vi "Omniax_mDrive_COM9_MM_BR.vi"() -> ()   [LabVIEW 2009]
uses:
  <vilib>/Instr/_visa.llb/VISA Configure Serial Port (Instr).vi
panel:
  out "Backlash corr":bool
  in  "Y Scan set":bool
  in  "Y Scan Velocity SP mm/sec":dbl
  in  "Y Scan Length SP mm":dbl
  in  "Y Move Set":bool
  out "Backlash steps/sec":i32
  out "Backlash":i32
  out "Y in Motion":bool
  in  "Reset":bool
  out "Reset Motor Step to":dbl
  in  "Reset Y Position to":dbl
  out "Y Velocity MV mm/sec":dbl
  in  "Y Velocity SP mm/sec":dbl
  in  "Y Position SP mm":dbl
  out "Y Position MV mm":dbl
  out "Holding Current %":i32
  out "Run Current %":i32
  out "Y Scan velocity MV mm/sec":dbl format="%#_6f"
  out "Y Scan length MV mm":dbl
  in  "Y Scan Cancel":bool
  out "Y Position mm PV":dbl
  out "offset":dbl
  out "mm/rev":dbl
  out "steps/rev":u32
  out "scan steps/secm return":i32
  in  "Y Scan Length SP steps":i32 min=-460800 max=460800 step=100
  out "Y Scan":bool
  in  "Y Scan Set":bool
  in  "Scan Go":bool
  in  "Y Velocity SP step/sec":i32
  in  "Y Scan Velocity SP steps/sec":i32=1 min=1 max=102400 step=1
  in  "Stop":bool
  out "Y in Range":bool
  out "Y Step PV":i32 max=2000
  out "Status":string
  in  "Go":bool
  in  "Y Step SP":i32=-20000 min=-460800 max=460800 step=500
  out "MINPOS":i32=-94296
  out "MAXPOS":i32=-34296
  out "COM PORT":refnum<visa-resource-name>="COM5"
  # "SY"
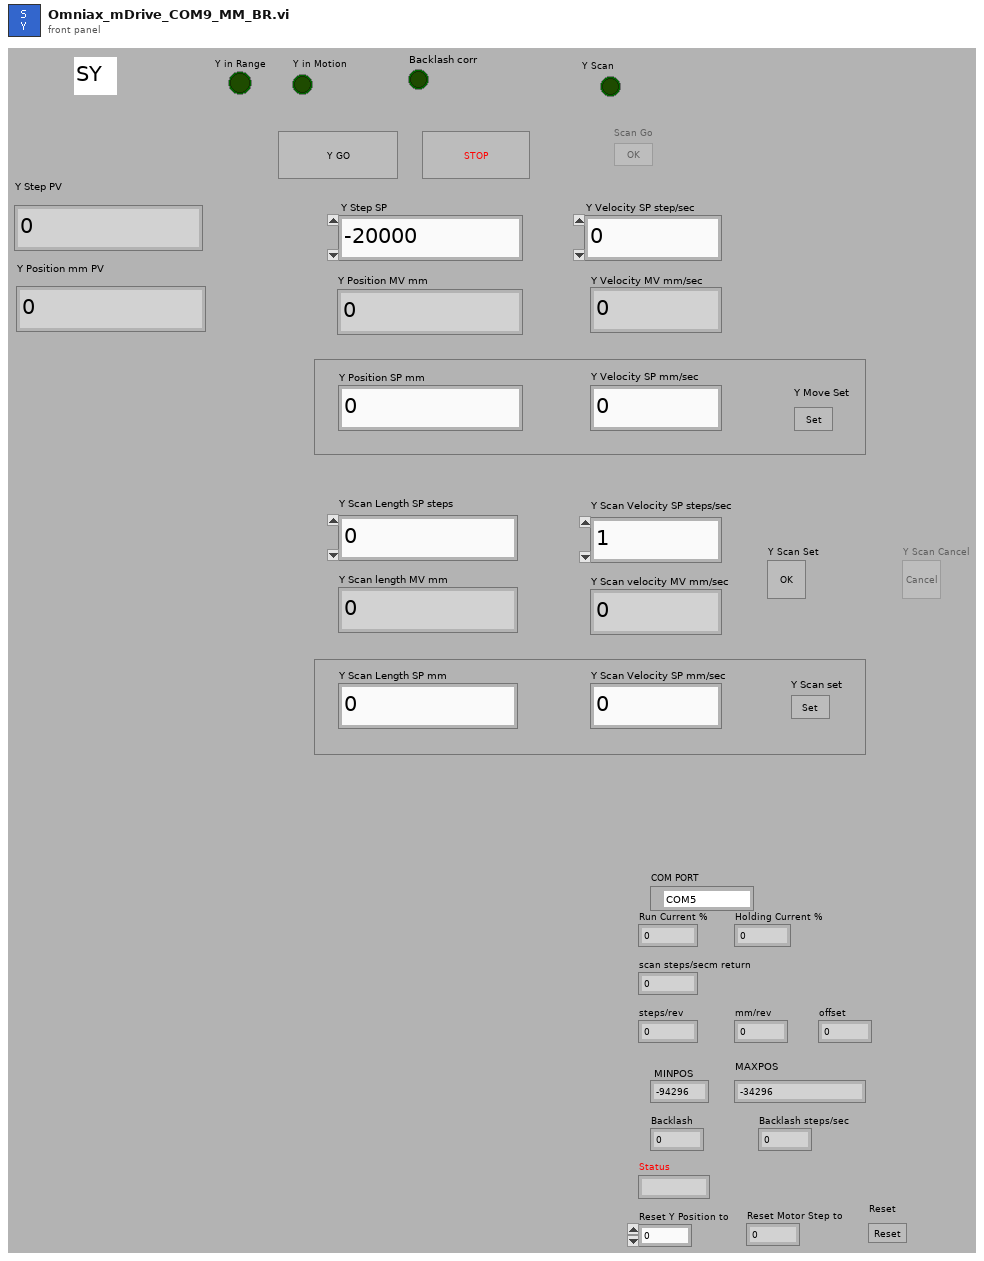
[diagram p1: front panel]
types:
  T1 = enum8{"Enabled", "Disabled", "Disabled and Grayed Out"}
  T2 = enum16{"Stop", "Reset", "Run Current", "Holding Current", "Accel Rate", "Decel Rate", "Move to Relative Position", "Move to Absolute Position", "Echo Mode", "Print Parameter", "Send String", "Microstep Resolution", "Set Current Position", "Max Velocity"}
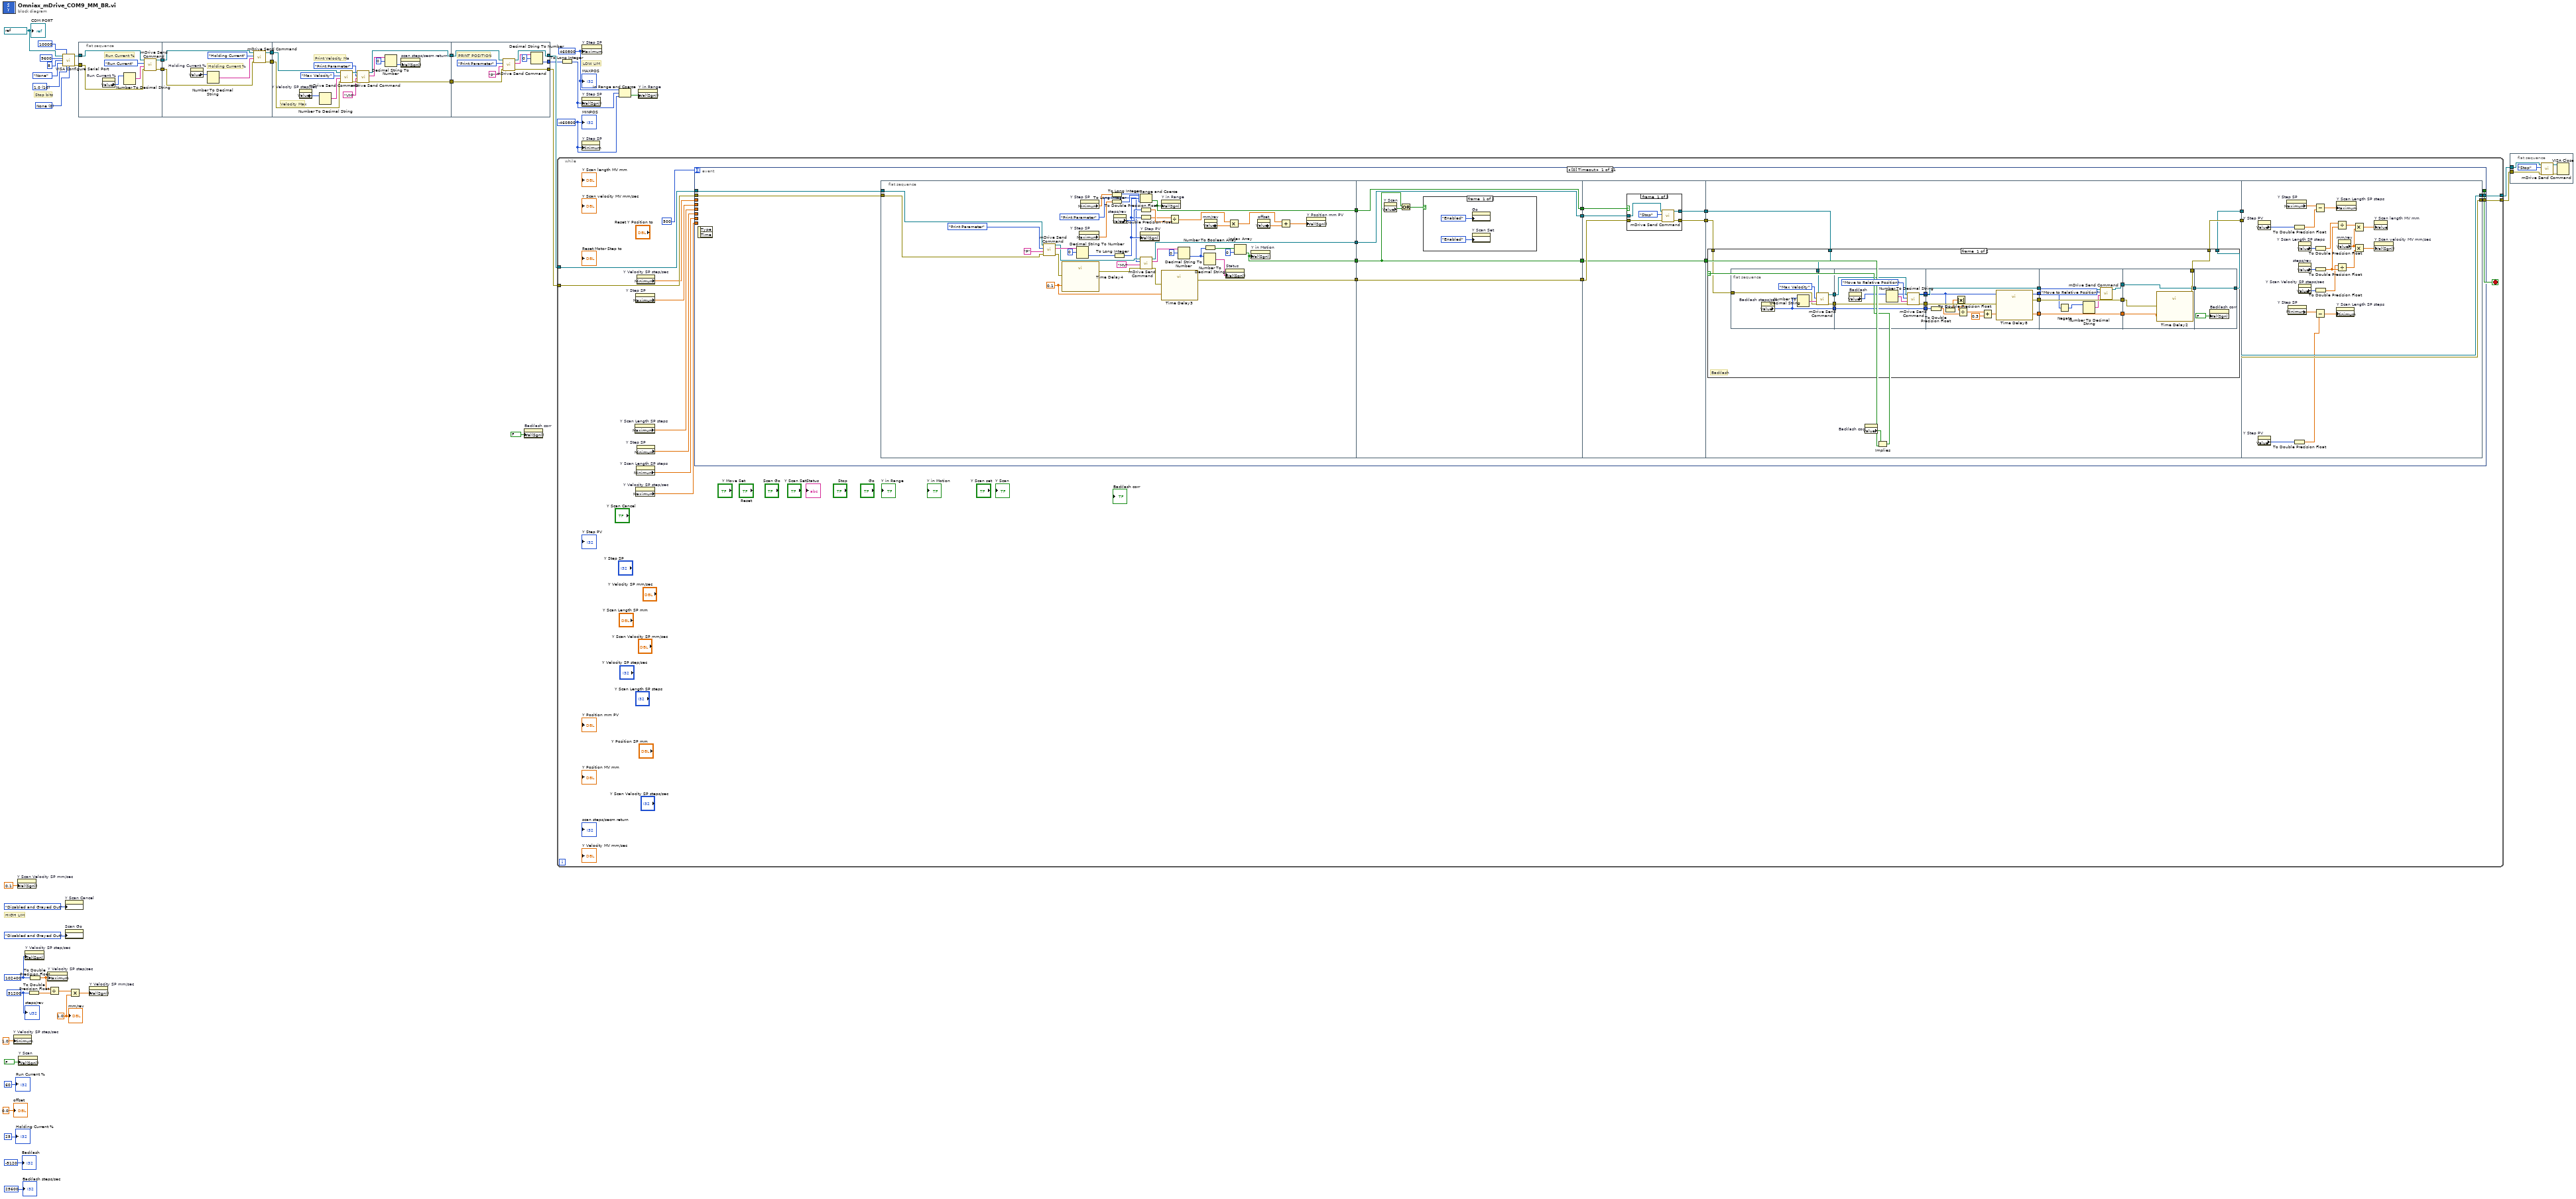
[diagram p0: block diagram]
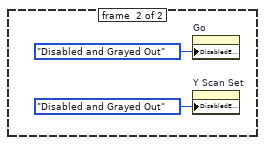
[diagram p2: hidden frame]
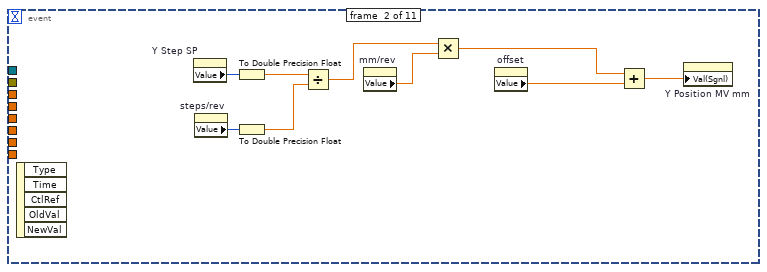
[diagram p5: hidden frame]
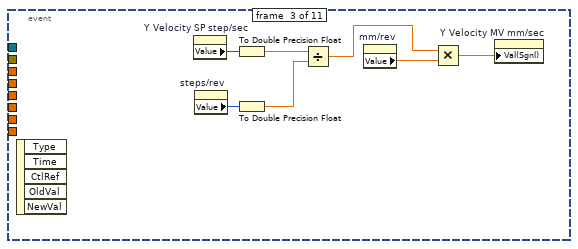
[diagram p6: hidden frame]
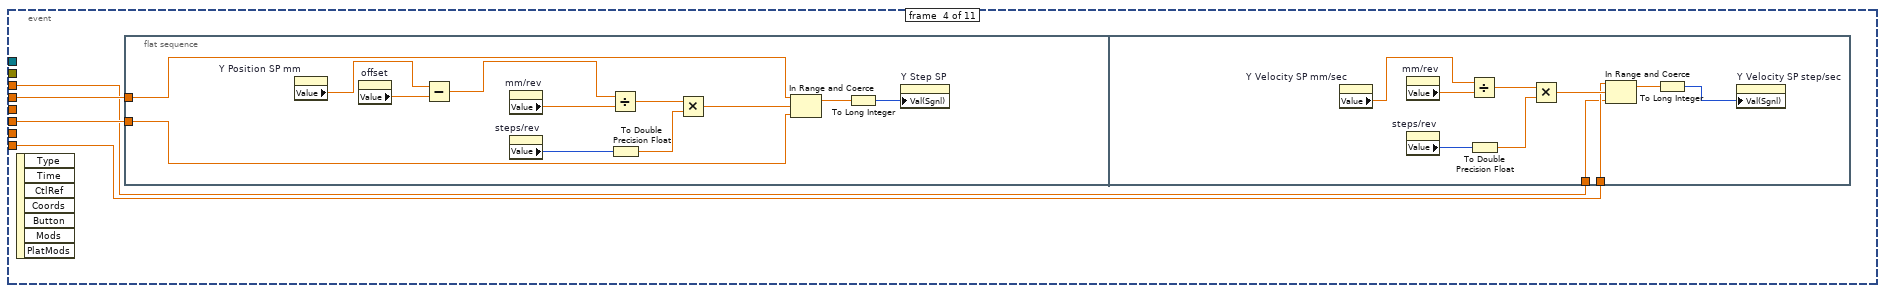
[diagram p7: hidden frame]
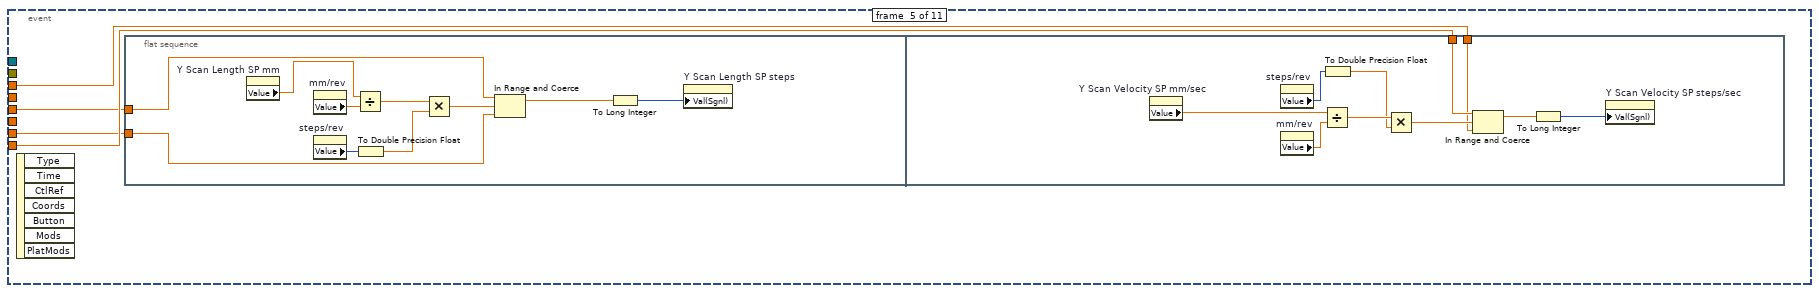
[diagram p8: hidden frame]
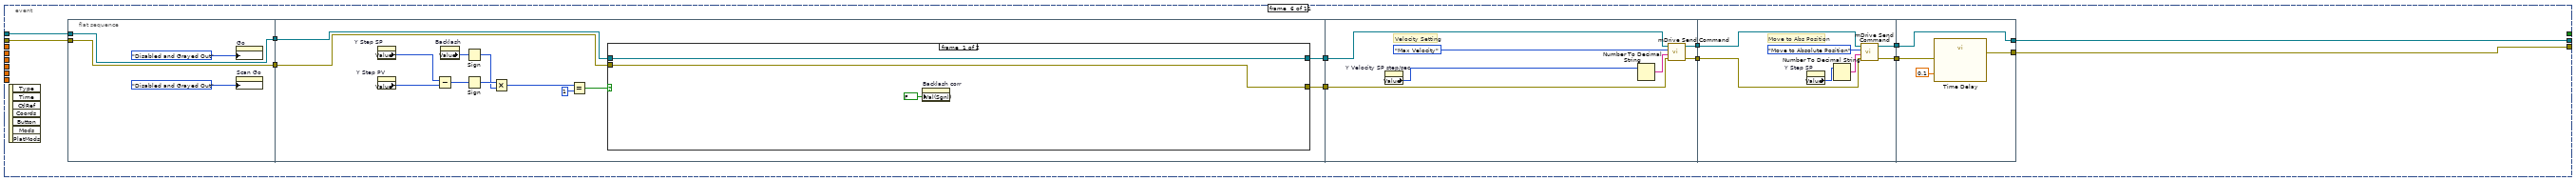
[diagram p9: hidden frame]
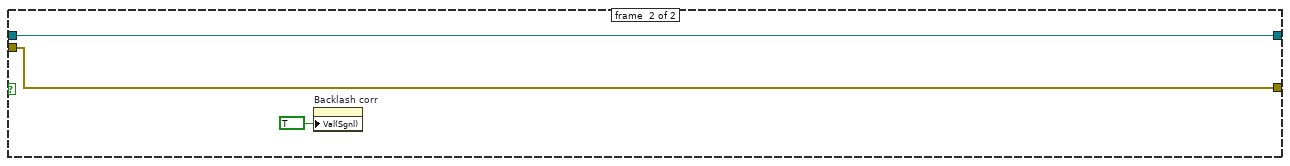
[diagram p10: hidden frame]
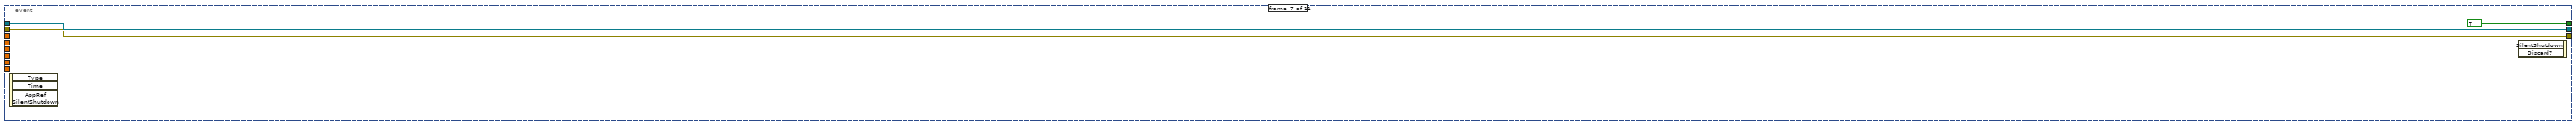
[diagram p11: hidden frame]
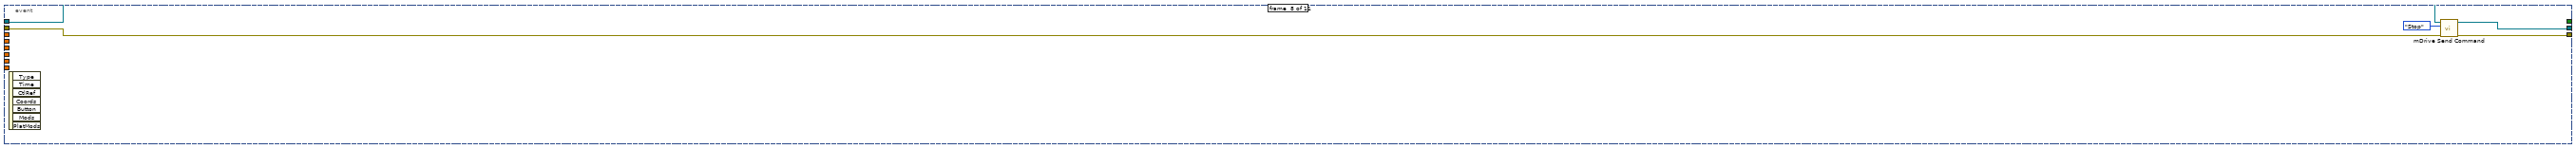
[diagram p12: hidden frame]
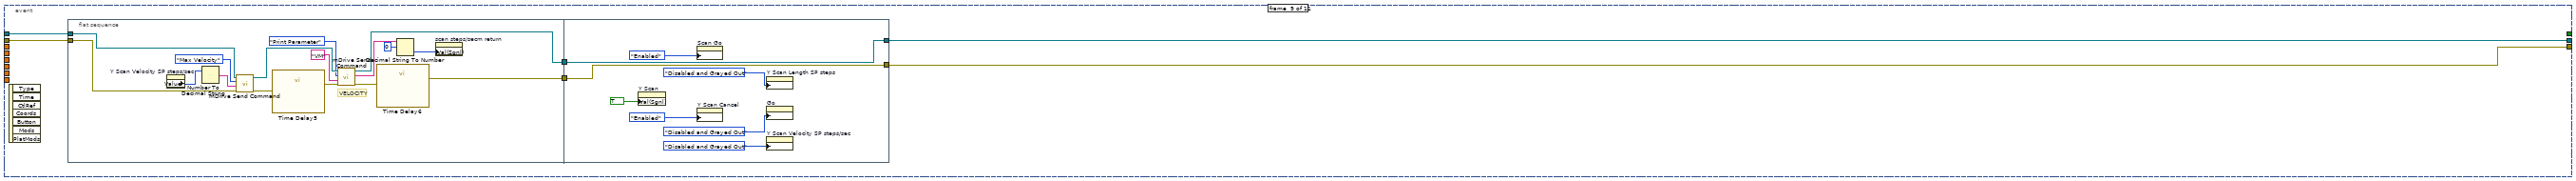
[diagram p13: hidden frame]
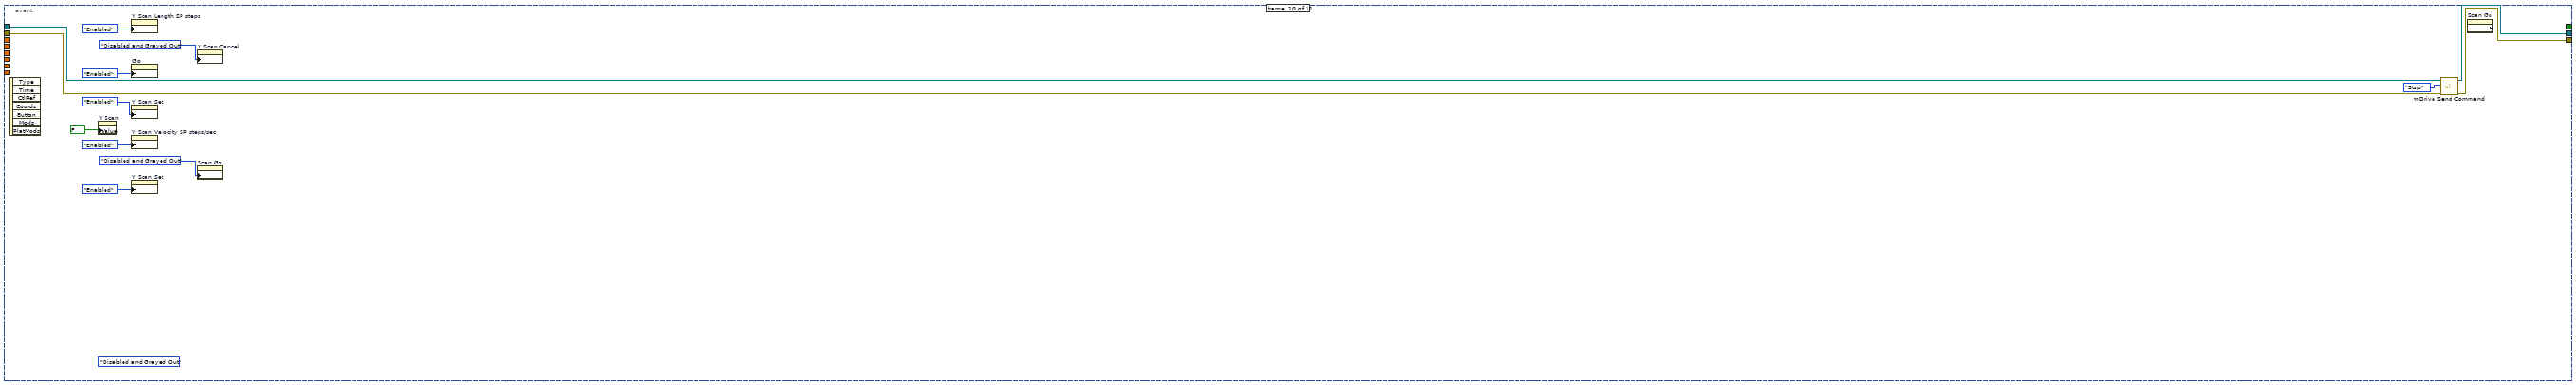
[diagram p14: hidden frame]
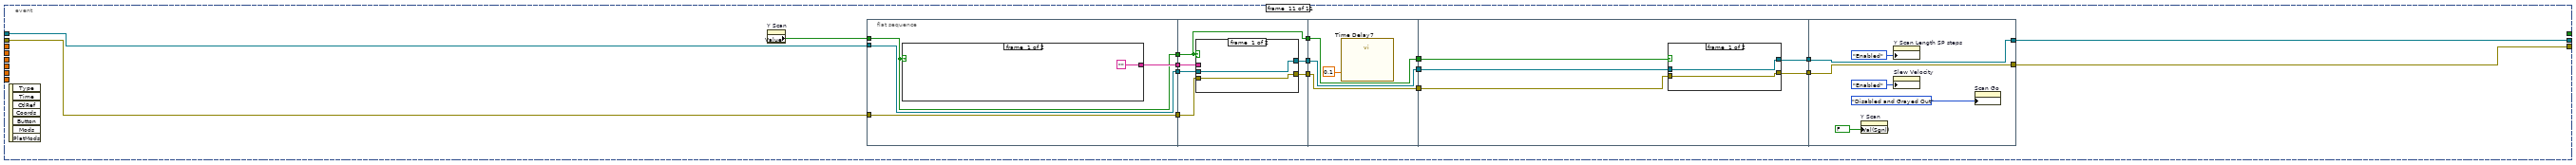
[diagram p15: hidden frame]
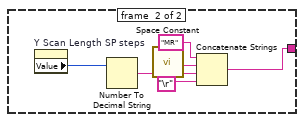
[diagram p16: hidden frame]
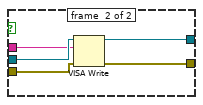
[diagram p17: hidden frame]
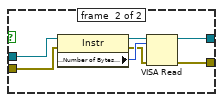
[diagram p18: hidden frame]
diagram:
  w7 = 1.0 ("MM/rev")
  w4 = u32 51200 ("step/rev")
  w9 = 102400 ("Value (Signaling)")
  w29 = -460800 ("lower limit")
  w28 = 460800 ("upper limit")
  w36 = refnum<visa-resource-name> "COM9" ("COM PORT")
  w38 = u16 0 items=["None", "XON/XOFF", "RTS/CTS", "XON/XOFF & RTS/CTS", "DTR/DSR", "XON/XOFF & DTR/DSR"] ("flow control (0:none)")
  w39 = u16 10 items=["1.0"=10, "1.5"=15, "2.0"=20] ("stop bits (10: 1 bit)")
  # "HIGH LIM"
  # "LOW LIM"
  # "Stop bits"
  n1 = property on="Y Velocity SP step/sec" class="DigNum (strict)"("Minimum"=1.0 ("Data Entry Limits:Minimum")) -> ()  [unwired: 2 in, 2 out]
  n2 = property on="Y Scan Velocity SP mm/sec" class="DigNum (strict)"("Val(Sgnl)"=0.1 ("Value (Signaling)")) -> ()  [unwired: 2 in, 2 out]
  n3 = property on="Y Scan" class="Bool (strict)"("Val(Sgnl)"=FALSE ("Value (Signaling)")) -> ()  [unwired: 2 in, 2 out]
  n4 = property on="Y Velocity SP step/sec" class="DigNum (strict)"("Val(Sgnl)"=w9) -> ()  [unwired: 2 in, 2 out]
  n5 = To Double Precision Float(number=w4) -> (double precision float=w5:dbl)
  n6 = To Double Precision Float(number=w9) -> (double precision float=w3:dbl)
  n7 = property on="Y Velocity SP step/sec" class="DigNum (strict)"("Maximum"=w3) -> ()  [unwired: 2 in, 2 out]
  n8 = Divide(x=w3, y=w5) -> (x/y=w8:dbl)
  n9 = call-poly "VISA Configure Serial Port"("VISA resource name"=w36, "timeout (10sec)"=u32 10000, "baud rate (9600)"=u32 9600, "data bits (8)"=u16 8, "parity (0:none)"=enum16{"None", "Odd", "Even", "Mark", "Space"}."None", "stop bits (10: 1 bit)"=w39, "flow control (0:none)"=w38) -> ("VISA resource name out"=w24:refnum<visa-resource-name>, "error out"=w23:errorcluster)  [unwired: 7 in]
  n10 = property on="Y Scan Cancel" class="Bool"("DisabledEnum"=T1."Disabled and Grayed Out" ("Disabled")) -> ()  [unwired: 2 in, 2 out]
  n11 = property on="Scan Go" class="Bool"("DisabledEnum"=T1."Disabled and Grayed Out" ("Disabled")) -> ()  [unwired: 2 in, 2 out]
  n12 = Multiply(x=w8, y=w7) -> (x*y=w6:dbl)
  n13 = flat-sequence {
    tunnel: w23 -> [w49]
    tunnel: w24 -> [w47]
    tunnel: [w46] -> w18
    tunnel: [w48] -> w16
    tunnel: w18 -> [w56]
    tunnel: [w55] -> w17
    tunnel: w16 -> [w53]
    tunnel: [w54] -> w15
    tunnel: [w66] -> w26
    tunnel: [w67] -> w25
    tunnel: w17 -> [w65]
    tunnel: w15 -> [w64]
    tunnel: [w79] -> w35
    tunnel: [w78] -> w34
    tunnel: [w73] -> w27
    tunnel: w26 -> [w77]
    tunnel: w25 -> [w76]
    frame #0 {
      # "Run Current %"
      n14 = property on="Run Current %" class="DigNum (strict)"() -> ("Value"=w44:i32)  [unwired: 2 in, 2 out]
      n15 = Number To Decimal String(number=w44) -> (decimal integer string=w45:string)  [unwired: 1 in]
      n16 = call "mDrive Send Command.vi"("error in (no error)"=w49, "Extra"=w45, "Command"=T2."Run Current", "VISA resource name"=w47) -> ("error out"=w48:errorcluster, "VISA resource name out"=w46:refnum<visa-resource-name>)  [unwired: 3 in, 1 out]
    }
    frame #1 {
      # "Holding Current %"
      n17 = property on="Holding Current %" class="DigNum (strict)"() -> ("Value"=w51:i32)  [unwired: 2 in, 2 out]
      n18 = Number To Decimal String(number=w51) -> (decimal integer string=w52:string)  [unwired: 1 in]
      n19 = call "mDrive Send Command.vi"("error in (no error)"=w53, "Extra"=w52, "Command"=T2."Holding Current", "VISA resource name"=w56) -> ("error out"=w54:errorcluster, "VISA resource name out"=w55:refnum<visa-resource-name>)  [unwired: 3 in, 1 out]
    }
    frame #2 {
      # "Print Velocity Ma"
      # "Velocity Max"
      n20 = property on="Y Velocity SP step/sec" class="DigNum (strict)"() -> ("Value"=w63:i32)  [unwired: 2 in, 2 out]
      n21 = Number To Decimal String(number=w63) -> (decimal integer string=w62:string)  [unwired: 1 in]
      n22 = call "mDrive Send Command.vi"("error in (no error)"=w64, "Extra"=w62, "Command"=T2."Max Velocity", "VISA resource name"=w65) -> ("error out"=w60:errorcluster, "VISA resource name out"=w70:refnum<visa-resource-name>)  [unwired: 3 in, 1 out]
      n23 = call "mDrive Send Command.vi"("error in (no error)"=w60, "Extra"="VM", "Command"=T2."Print Parameter", "VISA resource name"=w70) -> ("error out"=w67:errorcluster, "read buffer"=w68:string, "VISA resource name out"=w66:refnum<visa-resource-name>)  [unwired: 3 in]
      n24 = Decimal String To Number(string=w68, offset=0) -> (number=w61:i32)  [unwired: 1 in, 1 out]
      n25 = property on="scan steps/secm return" class="DigNum (strict)"("Val(Sgnl)"=w61) -> ()  [unwired: 2 in, 2 out]
    }
    frame #3 {
      # "PRINT POSITION"
      n26 = call "mDrive Send Command.vi"("error in (no error)"=w76, "Extra"="P", "Command"=T2."Print Parameter", "VISA resource name"=w77) -> ("error out"=w78:errorcluster, "read buffer"=w75:string, "VISA resource name out"=w79:refnum<visa-resource-name>)  [unwired: 3 in]
      n27 = Decimal String To Number(string=w75, offset=0) -> (number=w73:i32)  [unwired: 1 in, 1 out]
    }
  }
  n28 = property on="Y Velocity SP mm/sec" class="DigNum (strict)"("Val(Sgnl)"=w6) -> ()  [unwired: 2 in, 2 out]
  n29 = property on="Backlash corr" class="Bool (strict)"("Val(Sgnl)"=FALSE ("Value (Signaling)")) -> ()  [unwired: 2 in, 2 out]
  n30 = while {
    tunnel: w35 -> [w87]
    tunnel: w34 -> [w90]
    tunnel: [w91] -> w31
    tunnel: [w89] -> w32
    stop <- w86 stop-if-true
    n31 = property on="Y Scan Length SP steps" class="DigNum (strict)"() -> ("Maximum"=w80:dbl)  [unwired: 2 in, 2 out]
    n32 = property on="Y Step SP" class="DigNum (strict)"() -> ("Maximum"=w84:dbl)  [unwired: 2 in, 2 out]
    n33 = property on="Y Velocity SP step/sec" class="DigNum (strict)"() -> ("Maximum"=w83:dbl)  [unwired: 2 in, 2 out]
    n34 = property on="Y Scan Length SP steps" class="DigNum (strict)"() -> ("Minimum"=w81:dbl)  [unwired: 2 in, 2 out]
    n35 = property on="Y Velocity SP step/sec" class="DigNum (strict)"() -> ("Minimum"=w82:dbl)  [unwired: 2 in, 2 out]
    n36 = property on="Y Step SP" class="DigNum (strict)"() -> ("Minimum"=w85:dbl)  [unwired: 2 in, 2 out]
    n37 = event shown="[0] Timeout" {
      selector: _ -> [_ _ _ _ _ _ _ _ _ _ _]
      dyn-events: _ -> [_ _ _ _ _ _ _ _ _ _ _]
      timeout: 500 -> [_ _ _ _ _ _ _ _ _ _ _]
      tunnel: w90 -> [w108 _ _ _ _ w328 w378 w383 w390 w420 w444]
      tunnel: [w107 _ _ _ _ w334 w378 w381 w388 w422 w441] -> w91
      tunnel: w87 -> [w105 _ _ _ _ w329 w379 w384 w389 w421 w443]
      tunnel: [w106 _ _ _ _ w335 w379 w382 w385 w423 w442] -> w89
      tunnel: [_ _ _ _ _ _ TRUE _ _ _ _] -> w86
      tunnel: w85 -> [_ _ _ w277 _ _ _ _ _ _ _]
      tunnel: w84 -> [_ _ _ w276 _ _ _ _ _ _ _]
      tunnel: w83 -> [_ _ _ w275 w303 _ _ _ _ _ _]
      tunnel: w82 -> [_ _ _ w274 w302 _ _ _ _ _ _]
      tunnel: w81 -> [_ _ _ _ w301 _ _ _ _ _ _]
      tunnel: w80 -> [_ _ _ _ w300 _ _ _ _ _ _]
      event #0 {
        n38 = event-data() -> ()  [unwired: 1 in, 2 out]
        n39 = flat-sequence {
          tunnel: w108 -> [w140]
          tunnel: w105 -> [w139]
          tunnel: [w145] -> w104
          tunnel: [w119] -> w102
          tunnel: [w132] -> w100
          tunnel: [w109] -> w98
          tunnel: w104 -> [w151]
          tunnel: [w151] -> w103
          tunnel: w102 -> [w150]
          tunnel: [w150] -> w101
          tunnel: w100 -> [w149]
          tunnel: [w149] -> w99
          tunnel: w98 -> [w146]
          tunnel: [w146] -> w93
          tunnel: w103 -> [w158]
          tunnel: [w159] -> w97
          tunnel: w101 -> [w161]
          tunnel: [w160] -> w96
          tunnel: w99 -> [w157]
          tunnel: [w156] -> w94
          tunnel: w93 -> [w156]
          tunnel: w97 -> [w171]
          tunnel: w96 -> [w172]
          tunnel: [w170] -> w95
          tunnel: w94 -> [w174]
          tunnel: [w169] -> w92
          tunnel: [w256] -> w107
          tunnel: [w257] -> w106
          tunnel: w95 -> [w256]
          tunnel: w92 -> [w257]
          frame #0 {
            w113 = 0.1 ("Delay Time (s)")
            n40 = call "mDrive Send Command.vi"("error in (no error)"=w140, "Extra"="P", "Command"=T2."Print Parameter", "VISA resource name"=w139) -> ("error out"=w138:errorcluster, "read buffer"=w144:string, "VISA resource name out"=w142:refnum<visa-resource-name>)  [unwired: 3 in]
            n41 = call "Time Delay4"("error in (no error)"=w138, "Delay Time (s)"=w113) -> ("error out"=w137:errorcluster)  [unwired: 9 in]
            n42 = Decimal String To Number(string=w144, offset=0) -> (number=w122:i32)  [unwired: 1 in, 1 out]
            n43 = property on="Y Step SP" class="DigNum (strict)"() -> ("Maximum"=w134:dbl)  [unwired: 2 in, 2 out]
            n44 = property on="Y Step SP" class="DigNum (strict)"() -> ("Minimum"=w136:dbl)  [unwired: 2 in, 2 out]
            n45 = To Long Integer(number=w136) -> (32bit integer=w135:i32)
            n46 = To Long Integer(number=w134) -> (32bit integer=w133:i32)
            n47 = To Long Integer(number=w122) -> (32bit integer=w124:i32)
            n48 = property on="steps/rev" class="DigNum (strict)"() -> ("Value"=w130:u32)  [unwired: 2 in, 2 out]
            n49 = In Range and Coerce(upper limit=w133, x=w124, lower limit=w135) -> (In Range?=w132:bool)  [unwired: 1 out]
            n50 = To Double Precision Float(number=w130) -> (double precision float=w131:dbl)
            n51 = To Double Precision Float(number=w124) -> (double precision float=w125:dbl)
            n52 = property on="Y Step PV" class="DigNum (strict)"("Val(Sgnl)"=w124) -> ()  [unwired: 2 in, 2 out]
            n53 = call "mDrive Send Command.vi"("error in (no error)"=w137, "Extra"="MV", "Command"=T2."Print Parameter", "VISA resource name"=w142) -> ("error out"=w141:errorcluster, "read buffer"=w120:string, "VISA resource name out"=w145:refnum<visa-resource-name>)  [unwired: 3 in]
            n54 = property on="Y in Range" class="Bool (strict)"("Val(Sgnl)"=w132) -> ()  [unwired: 2 in, 2 out]
            n55 = call "Time Delay3"("error in (no error)"=w141, "Delay Time (s)"=w113) -> ("error out"=w119:errorcluster)  [unwired: 9 in]
            n56 = Divide(x=w125, y=w131) -> (x/y=w129:dbl)
            n57 = Decimal String To Number(string=w120, offset=0 ("offset (0)")) -> (number=w112:i32)  [unwired: 1 in, 1 out]
            n58 = Number To Decimal String(number=w112) -> (decimal integer string=w118:string)  [unwired: 1 in]
            n59 = property on="mm/rev" class="DigNum (strict)"() -> ("Value"=w128:dbl)  [unwired: 2 in, 2 out]
            n60 = Number To Boolean Array(number=w112) -> (Boolean array=w111:bool[])
            n61 = property on="Status" class="Str"("Val(Sgnl)"=w118) -> ()  [unwired: 2 in, 2 out]
            n62 = Multiply(x=w129, y=w128) -> (x*y=w127:dbl)
            n63 = Index Array(array=w111, index=0) -> (element=w109:bool)
            n64 = property on="Y in Motion" class="Bool (strict)"("Val(Sgnl)"=w109) -> ()  [unwired: 2 in, 2 out]
            n65 = property on="offset" class="DigNum (strict)"() -> ("Value"=w126:dbl)  [unwired: 2 in, 2 out]
            n66 = Add(x=w127, y=w126) -> (x+y=w123:dbl)
            n67 = property on="Y Position mm PV" class="DigNum (strict)"("Val(Sgnl)"=w123) -> ()  [unwired: 2 in, 2 out]
          }
          frame #1 {
            n68 = property on="Y Scan" class="Bool (strict)"() -> ("Value"=w147:bool)  [unwired: 2 in, 2 out]
            n69 = Or(x=w146, y=w147) -> (x .or. y?=w148:bool)
            n70 = case shown="False" w148 {
              frame #0 {
                n71 = property on="Go" class="Bool"("DisabledEnum"=T1."Enabled" ("Disabled")) -> ()  [unwired: 2 in, 2 out]
                n72 = property on="Y Scan Set" class="Bool"("DisabledEnum"=T1."Enabled" ("Disabled")) -> ()  [unwired: 2 in, 2 out]
              }
              frame #1 {
                n73 = property on="Go" class="Bool"("DisabledEnum"=T1."Disabled and Grayed Out" ("Disabled")) -> ()  [unwired: 2 in, 2 out]
                n74 = property on="Y Scan Set" class="Bool"("DisabledEnum"=T1."Disabled and Grayed Out" ("Disabled")) -> ()  [unwired: 2 in, 2 out]
              }
            }
          }
          frame #2 {
            n75 = case shown="False" w157 {
              tunnel: w158 -> [w164 w168]
              tunnel: [w165 w168] -> w159
              tunnel: [w166 w167] -> w160
              tunnel: w161 -> [w163 w167]
              frame #0 {
                n76 = call "mDrive Send Command.vi"("error in (no error)"=w163, "Command"=T2."Stop", "VISA resource name"=w164) -> ("error out"=w166:errorcluster, "VISA resource name out"=w165:refnum<visa-resource-name>)  [unwired: 4 in, 1 out]
              }
              frame #1 {
              }
            }
          }
          frame #3 {
            n77 = property on="Backlash corr" class="Bool (strict)"() -> ("Value"=w175:bool)  [unwired: 2 in, 2 out]
            n78 = Implies(1:w174, 2:w175) -> (0:w173:bool)
            n79 = case shown="False" w173 {
              tunnel: w172 -> [w182 w235]
              tunnel: w171 -> [w181 w236]
              tunnel: [w180 w235] -> w170
              tunnel: [w179 w236] -> w169
              frame #0 {
                # "Backlash"
                n80 = flat-sequence {
                  tunnel: [w197] -> w194
                  tunnel: [w199] -> w193
                  tunnel: [w198] -> w192
                  tunnel: w182 -> [w196]
                  tunnel: w181 -> [w195]
                  tunnel: w194 -> [w207]
                  tunnel: [w207] -> w191
                  tunnel: w193 -> [w206]
                  tunnel: w192 -> [w205]
                  tunnel: [w204] -> w190
                  tunnel: [w203] -> w189
                  tunnel: [w202] -> w178
                  tunnel: w191 -> [w217]
                  tunnel: w190 -> [w216]
                  tunnel: w189 -> [w214]
                  tunnel: [w215] -> w188
                  tunnel: [w214] -> w187
                  tunnel: [w213] -> w184
                  tunnel: [w212] -> w183
                  tunnel: w178 -> [w212]
                  tunnel: w188 -> [w228]
                  tunnel: w187 -> [w221]
                  tunnel: [w228] -> w186
                  tunnel: [w227] -> w185
                  tunnel: w184 -> [w227]
                  tunnel: w183 -> [w223]
                  tunnel: [w222] -> w176
                  tunnel: w186 -> [w232]
                  tunnel: w185 -> [w231]
                  tunnel: [w230] -> w180
                  tunnel: [w229] -> w177
                  tunnel: w176 -> [w229]
                  tunnel: [w234] -> w179
                  tunnel: w177 -> [w234]
                  frame #0 {
                    n81 = property on="Backlash steps/sec" class="DigNum (strict)"() -> ("Value"=w197:i32)  [unwired: 2 in, 2 out]
                    n82 = Number To Decimal String(number=w197) -> (decimal integer string=w200:string)  [unwired: 1 in]
                    n83 = call "mDrive Send Command.vi"("error in (no error)"=w196, "Extra"=w200, "Command"=T2."Max Velocity", "VISA resource name"=w195) -> ("error out"=w198:errorcluster, "VISA resource name out"=w199:refnum<visa-resource-name>)  [unwired: 3 in, 1 out]
                  }
                  frame #1 {
                    n84 = property on="Backlash" class="DigNum (strict)"() -> ("Value"=w202:i32)  [unwired: 2 in, 2 out]
                    n85 = Number To Decimal String(number=w202) -> (decimal integer string=w208:string)  [unwired: 1 in]
                    n86 = call "mDrive Send Command.vi"("error in (no error)"=w205, "Extra"=w208, "Command"=T2."Move to Relative Position", "VISA resource name"=w206) -> ("error out"=w204:errorcluster, "VISA resource name out"=w203:refnum<visa-resource-name>)  [unwired: 3 in, 1 out]
                  }
                  frame #2 {
                    n87 = To Double Precision Float(number=w217) -> (double precision float=w219:dbl)
                    n88 = To Double Precision Float(number=w212) -> (double precision float=w210:dbl)
                    n89 = Absolute Value(x=w210) -> (abs(x)=w211:dbl)
                    n90 = Divide(x=w211, y=w219) -> (x/y=w220:dbl)
                    n91 = Add(x=w220, y=0.3) -> (x+y=w213:dbl)
                    n92 = call "Time Delay8"("error in (no error)"=w216, "Delay Time (s)"=w213) -> ("error out"=w215:errorcluster)  [unwired: 9 in]
                  }
                  frame #3 {
                    n93 = Negate(x=w223) -> (-x=w224:i32)
                    n94 = Number To Decimal String(number=w224) -> (decimal integer string=w225:string)  [unwired: 1 in]
                    n95 = call "mDrive Send Command.vi"("Extra"=w225, "Command"=T2."Move to Relative Position", "VISA resource name"=w221) -> ("VISA resource name out"=w222:refnum<visa-resource-name>)  [unwired: 4 in, 2 out]
                  }
                  frame #4 {
                    n96 = call "Time Delay2"("error in (no error)"=w232, "Delay Time (s)"=w231) -> ("error out"=w230:errorcluster)  [unwired: 9 in]
                  }
                  frame #5 {
                    n97 = property on="Backlash corr" class="Bool (strict)"("Val(Sgnl)"=FALSE ("Value (Signaling)")) -> ()  [unwired: 2 in, 2 out]
                  }
                }
              }
              frame #1 {
              }
            }
          }
          frame #4 {
            n98 = property on="Y Step PV" class="DigNum (strict)"() -> ("Value"=w246:i32)  [unwired: 2 in, 2 out]
            n99 = property on="Y Step PV" class="DigNum (strict)"() -> ("Value"=w244:i32)  [unwired: 2 in, 2 out]
            n100 = property on="Y Step SP" class="DigNum (strict)"() -> ("Maximum"=w253:dbl)  [unwired: 2 in, 2 out]
            n101 = property on="Y Step SP" class="DigNum (strict)"() -> ("Minimum"=w254:dbl)  [unwired: 2 in, 2 out]
            n102 = To Double Precision Float(number=w246) -> (double precision float=w245:dbl)
            n103 = To Double Precision Float(number=w244) -> (double precision float=w243:dbl)
            n104 = property on="Y Scan Velocity SP steps/sec" class="DigNum (strict)"() -> ("Value"=w241:i32)  [unwired: 2 in, 2 out]
            n105 = property on="Y Scan Length SP steps" class="DigNum (strict)"() -> ("Value"=w250:i32)  [unwired: 2 in, 2 out]
            n106 = property on="steps/rev" class="DigNum (strict)"() -> ("Value"=w248:u32)  [unwired: 2 in, 2 out]
            n107 = Subtract(x=w253, y=w245) -> (x-y=w252:dbl)
            n108 = Subtract(x=w254, y=w243) -> (x-y=w255:dbl)
            n109 = To Double Precision Float(number=w250) -> (double precision float=w249:dbl)
            n110 = To Double Precision Float(number=w248) -> (double precision float=w242:dbl)
            n111 = To Double Precision Float(number=w241) -> (double precision float=w240:dbl)
            n112 = property on="Y Scan Length SP steps" class="DigNum (strict)"("Maximum"=w252) -> ()  [unwired: 2 in, 2 out]
            n113 = Divide(x=w249, y=w242) -> (x/y=w251:dbl)
            n114 = Divide(x=w240, y=w242) -> (x/y=w239:dbl)
            n115 = property on="Y Scan Length SP steps" class="DigNum (strict)"("Minimum"=w255) -> ()  [unwired: 2 in, 2 out]
            n116 = property on="mm/rev" class="DigNum (strict)"() -> ("Value"=w247:dbl)  [unwired: 2 in, 2 out]
            n117 = Multiply(x=w251, y=w247) -> (x*y=w238:dbl)
            n118 = Multiply(x=w247, y=w239) -> (x*y=w237:dbl)
            n119 = property on="Y Scan length MV mm" class="DigNum (strict)"("Value"=w238) -> ()  [unwired: 2 in, 2 out]
            n120 = property on="Y Scan velocity MV mm/sec" class="DigNum (strict)"("Val(Sgnl)"=w237) -> ()  [unwired: 2 in, 2 out]
          }
        }
      }
      event #1 {
        n121 = event-data() -> ()  [unwired: 1 in, 5 out]
        n122 = property on="Y Step SP" class="DigNum (strict)"() -> ("Value"=w259:i32)  [unwired: 2 in, 2 out]
        n123 = property on="steps/rev" class="DigNum (strict)"() -> ("Value"=w260:u32)  [unwired: 2 in, 2 out]
        n124 = To Double Precision Float(number=w259) -> (double precision float=w261:dbl)
        n125 = To Double Precision Float(number=w260) -> (double precision float=w266:dbl)
        n126 = Divide(x=w261, y=w266) -> (x/y=w265:dbl)
        n127 = property on="mm/rev" class="DigNum (strict)"() -> ("Value"=w264:dbl)  [unwired: 2 in, 2 out]
        n128 = Multiply(x=w265, y=w264) -> (x*y=w263:dbl)
        n129 = property on="offset" class="DigNum (strict)"() -> ("Value"=w262:dbl)  [unwired: 2 in, 2 out]
        n130 = Add(x=w263, y=w262) -> (x+y=w258:dbl)
        n131 = property on="Y Position MV mm" class="DigNum (strict)"("Val(Sgnl)"=w258) -> ()  [unwired: 2 in, 2 out]
      }
      event #2 {
        n132 = event-data() -> ()  [unwired: 1 in, 5 out]
        n133 = property on="Y Velocity SP step/sec" class="DigNum (strict)"() -> ("Value"=w268:i32)  [unwired: 2 in, 2 out]
        n134 = property on="steps/rev" class="DigNum (strict)"() -> ("Value"=w269:u32)  [unwired: 2 in, 2 out]
        n135 = To Double Precision Float(number=w268) -> (double precision float=w270:dbl)
        n136 = To Double Precision Float(number=w269) -> (double precision float=w273:dbl)
        n137 = Divide(x=w270, y=w273) -> (x/y=w272:dbl)
        n138 = property on="mm/rev" class="DigNum (strict)"() -> ("Value"=w271:dbl)  [unwired: 2 in, 2 out]
        n139 = Multiply(x=w272, y=w271) -> (x*y=w267:dbl)
        n140 = property on="Y Velocity MV mm/sec" class="DigNum (strict)"("Val(Sgnl)"=w267) -> ()  [unwired: 2 in, 2 out]
      }
      event #3 {
        n141 = event-data() -> ()  [unwired: 1 in, 7 out]
        n142 = flat-sequence {
          tunnel: w277 -> [w280]
          tunnel: w276 -> [w279]
          tunnel: w275 -> [w292]
          tunnel: w274 -> [w291]
          frame #0 {
            n143 = property on="Y Position SP mm" class="DigNum (strict)"() -> ("Value"=w282:dbl)  [unwired: 2 in, 2 out]
            n144 = property on="offset" class="DigNum (strict)"() -> ("Value"=w283:dbl)  [unwired: 2 in, 2 out]
            n145 = Subtract(x=w282, y=w283) -> (x-y=w287:dbl)
            n146 = property on="mm/rev" class="DigNum (strict)"() -> ("Value"=w286:dbl)  [unwired: 2 in, 2 out]
            n147 = property on="steps/rev" class="DigNum (strict)"() -> ("Value"=w285:u32)  [unwired: 2 in, 2 out]
            n148 = Divide(x=w287, y=w286) -> (x/y=w288:dbl)
            n149 = To Double Precision Float(number=w285) -> (double precision float=w289:dbl)
            n150 = Multiply(x=w288, y=w289) -> (x*y=w281:dbl)
            n151 = In Range and Coerce(upper limit=w279, x=w281, lower limit=w280) -> (coerced(x)=w278:dbl)  [unwired: 1 out]
            n152 = To Long Integer(number=w278) -> (32bit integer=w284:i32)
            n153 = property on="Y Step SP" class="DigNum (strict)"("Val(Sgnl)"=w284) -> ()  [unwired: 2 in, 2 out]
          }
          frame #1 {
            n154 = property on="Y Velocity SP mm/sec" class="DigNum (strict)"() -> ("Value"=w297:dbl)  [unwired: 2 in, 2 out]
            n155 = property on="mm/rev" class="DigNum (strict)"() -> ("Value"=w299:dbl)  [unwired: 2 in, 2 out]
            n156 = property on="steps/rev" class="DigNum (strict)"() -> ("Value"=w295:u32)  [unwired: 2 in, 2 out]
            n157 = Divide(x=w297, y=w299) -> (x/y=w298:dbl)
            n158 = To Double Precision Float(number=w295) -> (double precision float=w296:dbl)
            n159 = Multiply(x=w298, y=w296) -> (x*y=w293:dbl)
            n160 = In Range and Coerce(upper limit=w292, x=w293, lower limit=w291) -> (coerced(x)=w290:dbl)  [unwired: 1 out]
            n161 = To Long Integer(number=w290) -> (32bit integer=w294:i32)
            n162 = property on="Y Velocity SP step/sec" class="DigNum (strict)"("Val(Sgnl)"=w294) -> ()  [unwired: 2 in, 2 out]
          }
        }
      }
      event #4 {
        n163 = event-data() -> ()  [unwired: 1 in, 7 out]
        n164 = flat-sequence {
          tunnel: w301 -> [w305]
          tunnel: w300 -> [w304]
          tunnel: w303 -> [w315]
          tunnel: w302 -> [w314]
          frame #0 {
            n165 = property on="Y Scan Length SP mm" class="DigNum (strict)"() -> ("Value"=w308:dbl)  [unwired: 2 in, 2 out]
            n166 = property on="mm/rev" class="DigNum (strict)"() -> ("Value"=w311:dbl)  [unwired: 2 in, 2 out]
            n167 = property on="steps/rev" class="DigNum (strict)"() -> ("Value"=w310:u32)  [unwired: 2 in, 2 out]
            n168 = Divide(x=w308, y=w311) -> (x/y=w312:dbl)
            n169 = To Double Precision Float(number=w310) -> (double precision float=w313:dbl)
            n170 = Multiply(x=w312, y=w313) -> (x*y=w307:dbl)
            n171 = In Range and Coerce(upper limit=w304, x=w307, lower limit=w305) -> (coerced(x)=w306:dbl)  [unwired: 1 out]
            n172 = To Long Integer(number=w306) -> (32bit integer=w309:i32)
            n173 = property on="Y Scan Length SP steps" class="DigNum (strict)"("Val(Sgnl)"=w309) -> ()  [unwired: 2 in, 2 out]
          }
          frame #1 {
            n174 = property on="Y Scan Velocity SP mm/sec" class="DigNum (strict)"() -> ("Value"=w321:dbl)  [unwired: 2 in, 2 out]
            n175 = property on="steps/rev" class="DigNum (strict)"() -> ("Value"=w319:u32)  [unwired: 2 in, 2 out]
            n176 = property on="mm/rev" class="DigNum (strict)"() -> ("Value"=w323:dbl)  [unwired: 2 in, 2 out]
            n177 = Divide(x=w321, y=w323) -> (x/y=w322:dbl)
            n178 = To Double Precision Float(number=w319) -> (double precision float=w320:dbl)
            n179 = Multiply(x=w322, y=w320) -> (x*y=w317:dbl)
            n180 = In Range and Coerce(upper limit=w315, x=w317, lower limit=w314) -> (coerced(x)=w316:dbl)  [unwired: 1 out]
            n181 = To Long Integer(number=w316) -> (32bit integer=w318:i32)
            n182 = property on="Y Scan Velocity SP steps/sec" class="DigNum (strict)"("Val(Sgnl)"=w318) -> ()  [unwired: 2 in, 2 out]
          }
        }
      }
      event #5 {
        n183 = event-data() -> ()  [unwired: 1 in, 7 out]
        n184 = flat-sequence {
          tunnel: w328 -> [w338]
          tunnel: w329 -> [w339]
          tunnel: [w339] -> w325
          tunnel: [w338] -> w324
          tunnel: [w342] -> w327
          tunnel: [w341] -> w326
          tunnel: w325 -> [w344]
          tunnel: w324 -> [w343]
          tunnel: [w362] -> w331
          tunnel: [w361] -> w330
          tunnel: w327 -> [w360]
          tunnel: w326 -> [w359]
          tunnel: [w369] -> w333
          tunnel: [w368] -> w332
          tunnel: w331 -> [w367]
          tunnel: w330 -> [w366]
          tunnel: [w375] -> w334
          tunnel: [w376] -> w335
          tunnel: w333 -> [w376]
          tunnel: w332 -> [w374]
          frame #0 {
            n185 = property on="Go" class="Bool"("DisabledEnum"=T1."Disabled and Grayed Out" ("Disabled")) -> ()  [unwired: 2 in, 2 out]
            n186 = property on="Scan Go" class="Bool"("DisabledEnum"=T1."Disabled and Grayed Out" ("Disabled")) -> ()  [unwired: 2 in, 2 out]
          }
          frame #1 {
            n187 = property on="Y Step SP" class="DigNum (strict)"() -> ("Value"=w352:i32)  [unwired: 2 in, 2 out]
            n188 = property on="Y Step PV" class="DigNum (strict)"() -> ("Value"=w351:i32)  [unwired: 2 in, 2 out]
            n189 = Subtract(x=w352, y=w351) -> (x-y=w350:i32)
            n190 = property on="Backlash" class="DigNum (strict)"() -> ("Value"=w340:i32)  [unwired: 2 in, 2 out]
            n191 = Sign(1:w340) -> (0:w348:i32)
            n192 = Sign(1:w350) -> (0:w349:i32)
            n193 = Multiply(x=w349, y=w348) -> (x*y=w347:i32)
            n194 = Equal?(x=w347, y=1) -> (x = y?=w345:bool)
            n195 = case shown="False" w345 {
              tunnel: w344 -> [w355 w357]
              tunnel: w343 -> [w354 w356]
              tunnel: [w354 w356] -> w342
              tunnel: [w355 w357] -> w341
              frame #0 {
                n196 = property on="Backlash corr" class="Bool (strict)"("Val(Sgnl)"=FALSE ("Value (Signaling)")) -> ()  [unwired: 2 in, 2 out]
              }
              frame #1 {
                n197 = property on="Backlash corr" class="Bool (strict)"("Val(Sgnl)"=TRUE ("Value (Signaling)")) -> ()  [unwired: 2 in, 2 out]
              }
            }
          }
          frame #2 {
            # "Velocity Setting"
            n198 = property on="Y Velocity SP step/sec" class="DigNum (strict)"() -> ("Value"=w363:i32)  [unwired: 2 in, 2 out]
            n199 = Number To Decimal String(number=w363) -> (decimal integer string=w364:string)  [unwired: 1 in]
            n200 = call "mDrive Send Command.vi"("error in (no error)"=w360, "Extra"=w364, "Command"=T2."Max Velocity", "VISA resource name"=w359) -> ("error out"=w361:errorcluster, "VISA resource name out"=w362:refnum<visa-resource-name>)  [unwired: 3 in, 1 out]
          }
          frame #3 {
            # "Move to Abs Position"
            n201 = property on="Y Step SP" class="DigNum (strict)"() -> ("Value"=w372:i32)  [unwired: 2 in, 2 out]
            n202 = Number To Decimal String(number=w372) -> (decimal integer string=w371:string)  [unwired: 1 in]
            n203 = call "mDrive Send Command.vi"("error in (no error)"=w366, "Extra"=w371, "Command"=T2."Move to Absolute Position", "VISA resource name"=w367) -> ("error out"=w368:errorcluster, "VISA resource name out"=w369:refnum<visa-resource-name>)  [unwired: 3 in, 1 out]
          }
          frame #4 {
            n204 = call "Time Delay"("error in (no error)"=w374, "Delay Time (s)"=0.1) -> ("error out"=w375:errorcluster)  [unwired: 9 in]
          }
        }
      }
      event #6 {
        n205 = event-data() -> ()  [unwired: 1 in, 4 out]
        n206 = event-data() -> ()  [unwired: 3 in, 1 out]
      }
      event #7 {
        n207 = event-data() -> ()  [unwired: 1 in, 7 out]
        n208 = call "mDrive Send Command.vi"("error in (no error)"=w383, "Command"=T2."Stop", "VISA resource name"=w384) -> ("error out"=w381:errorcluster, "VISA resource name out"=w382:refnum<visa-resource-name>)  [unwired: 4 in, 1 out]
      }
      event #8 {
        n209 = event-data() -> ()  [unwired: 1 in, 7 out]
        n210 = flat-sequence {
          tunnel: w390 -> [w400]
          tunnel: w389 -> [w399]
          tunnel: [w396] -> w387
          tunnel: [w394] -> w386
          tunnel: [w413] -> w388
          tunnel: [w414] -> w385
          tunnel: w387 -> [w414]
          tunnel: w386 -> [w413]
          frame #0 {
            # "VELOCITY"
            n211 = property on="Y Scan Velocity SP steps/sec" class="DigNum (strict)"() -> ("Value"=w397:i32)  [unwired: 2 in, 2 out]
            n212 = Number To Decimal String(number=w397) -> (decimal integer string=w398:string)  [unwired: 1 in]
            n213 = call "mDrive Send Command.vi"("error in (no error)"=w400, "Extra"=w398, "Command"=T2."Max Velocity", "VISA resource name"=w399) -> ("error out"=w401:errorcluster, "VISA resource name out"=w406:refnum<visa-resource-name>)  [unwired: 3 in, 1 out]
            n214 = call "Time Delay5"("error in (no error)"=w401) -> ("error out"=w404:errorcluster)  [unwired: 10 in]
            n215 = call "mDrive Send Command.vi"("error in (no error)"=w404, "Extra"="VM", "Command"=T2."Print Parameter", "VISA resource name"=w406) -> ("error out"=w395:errorcluster, "read buffer"=w402:string, "VISA resource name out"=w396:refnum<visa-resource-name>)  [unwired: 3 in]
            n216 = call "Time Delay6"("error in (no error)"=w395) -> ("error out"=w394:errorcluster)  [unwired: 10 in]
            n217 = Decimal String To Number(string=w402, offset=0) -> (number=w405:i32)  [unwired: 1 in, 1 out]
            n218 = property on="scan steps/secm return" class="DigNum (strict)"("Val(Sgnl)"=w405) -> ()  [unwired: 2 in, 2 out]
          }
          frame #1 {
            n219 = property on="Y Scan" class="Bool (strict)"("Val(Sgnl)"=TRUE ("Slew Ready 2")) -> ()  [unwired: 2 in, 2 out]
            n220 = property on="Scan Go" class="Bool"("DisabledEnum"=T1."Enabled" ("Disabled")) -> ()  [unwired: 2 in, 2 out]
            n221 = property on="Y Scan Cancel" class="Bool"("DisabledEnum"=T1."Enabled" ("Disabled")) -> ()  [unwired: 2 in, 2 out]
            n222 = property on="Y Scan Length SP steps" class="DigNum (strict)"("DisabledEnum"=T1."Disabled and Grayed Out" ("Disabled")) -> ()  [unwired: 2 in, 2 out]
            n223 = property on="Go" class="Bool"("DisabledEnum"=T1."Disabled and Grayed Out" ("Disabled")) -> ()  [unwired: 2 in, 2 out]
            n224 = property on="Y Scan Velocity SP steps/sec" class="DigNum (strict)"("DisabledEnum"=T1."Disabled and Grayed Out" ("Disabled")) -> ()  [unwired: 2 in, 2 out]
          }
        }
      }
      event #9 {
        (unwired) T1."Disabled and Grayed Out" ("Disabled")
        n225 = event-data() -> ()  [unwired: 1 in, 7 out]
        n226 = property on="Y Scan" class="Bool (strict)"("Value"=FALSE ("Slew Ready")) -> ()  [unwired: 2 in, 2 out]
        n227 = property on="Y Scan Length SP steps" class="DigNum (strict)"("DisabledEnum"=T1."Enabled" ("Disabled")) -> ()  [unwired: 2 in, 2 out]
        n228 = property on="Go" class="Bool"("DisabledEnum"=T1."Enabled" ("Disabled")) -> ()  [unwired: 2 in, 2 out]
        n229 = property on="Y Scan Set" class="Bool"("DisabledEnum"=T1."Enabled" ("Disabled")) -> ()  [unwired: 2 in, 2 out]
        n230 = property on="Y Scan Velocity SP steps/sec" class="DigNum (strict)"("DisabledEnum"=T1."Enabled" ("Disabled")) -> ()  [unwired: 2 in, 2 out]
        n231 = property on="Y Scan Set" class="Bool"("DisabledEnum"=T1."Enabled" ("Disabled")) -> ()  [unwired: 2 in, 2 out]
        n232 = property on="Y Scan Cancel" class="Bool"("DisabledEnum"=T1."Disabled and Grayed Out" ("Disabled")) -> ()  [unwired: 2 in, 2 out]
        n233 = property on="Scan Go" class="Bool"("DisabledEnum"=T1."Disabled and Grayed Out" ("Disabled")) -> ()  [unwired: 2 in, 2 out]
        n234 = call "mDrive Send Command.vi"("error in (no error)"=w420, "Command"=T2."Stop", "VISA resource name"=w421) -> ("error out"=w422:errorcluster, "VISA resource name out"=w423:refnum<visa-resource-name>)  [unwired: 4 in, 1 out]
        n235 = property on="Scan Go" class="Bool" props=["DisabledEnum"]() -> ()  [unwired: 2 in, 3 out]
      }
      event #10 {
        n236 = event-data() -> ()  [unwired: 1 in, 7 out]
        n237 = property on="Y Scan" class="Bool (strict)"() -> ("Value"=w431:bool)  [unwired: 2 in, 2 out]
        n238 = flat-sequence {
          tunnel: w444 -> [w447]
          tunnel: w443 -> [w448]
          tunnel: [w448] -> w440
          tunnel: [w447] -> w439
          tunnel: [w446] -> w438
          tunnel: w431 -> [w445]
          tunnel: [w445] -> w430
          tunnel: w440 -> [w459]
          tunnel: [w461] -> w435
          tunnel: w439 -> [w458]
          tunnel: [w460] -> w433
          tunnel: w438 -> [w457]
          tunnel: w430 -> [w456]
          tunnel: [w456] -> w428
          tunnel: w435 -> [w472]
          tunnel: [w472] -> w434
          tunnel: w433 -> [w471]
          tunnel: [w471] -> w432
          tunnel: [w469] -> w429
          tunnel: w428 -> [w469]
          tunnel: w434 -> [w477]
          tunnel: [w475] -> w437
          tunnel: w432 -> [w476]
          tunnel: [w474] -> w436
          tunnel: w429 -> [w473]
          tunnel: w437 -> [w492]
          tunnel: w436 -> [w491]
          tunnel: [w492] -> w442
          tunnel: [w491] -> w441
          frame #0 {
            n239 = case shown="True" w445 {
              tunnel: ["" w450] -> w446
              frame #0 {
              }
              frame #1 {
                n240 = property on="Y Scan Length SP steps" class="DigNum (strict)"() -> ("Value"=w455:i32)  [unwired: 2 in, 2 out]
                n241 = Number To Decimal String(number=w455) -> (decimal integer string=w452:string)  [unwired: 1 in]
                n242 = call <vilib>:"Space Constant.vi"() -> ("String"=w453:string)
                n243 = Concatenate Strings("MR", w453, w452, "\r") -> (w450:string)
              }
            }
          }
          frame #1 {
            n244 = case shown="True" w456 {
              tunnel: [w463 w468] -> w461
              tunnel: [w462 w467] -> w460
              tunnel: w459 -> [w463 w466]
              tunnel: w458 -> [w462 w465]
              tunnel: w457 -> [_ w464]
              frame #0 {
              }
              frame #1 {
                n245 = VISA Write(VISA resource name=w466, write buffer=w464, error in (no error)=w465) -> (VISA resource name out=w468:refnum<visa-resource-name>, error out=w467:errorcluster)  [unwired: 1 out]
              }
            }
          }
          frame #2 {
            n246 = call "Time Delay7"("Delay Time (s)"=0.1) -> ()  [unwired: 10 in, 1 out]
          }
          frame #3 {
            n247 = case shown="True" w473 {
              tunnel: w477 -> [w479 w483]
              tunnel: w476 -> [w478 w482]
              tunnel: [w479 w481] -> w475
              tunnel: [w478 w480] -> w474
              frame #0 {
              }
              frame #1 {
                n248 = property class="Instr"(reference=w483, error in=w482) -> (reference out=w485:refnum<visa-resource-name>, error out=w484:errorcluster, "Serial Settings:Number of Bytes at Serial Port"=w486:u32)
                n249 = VISA Read(VISA resource name=w485, byte count=w486, error in (no error)=w484) -> (VISA resource name out=w481:refnum<visa-resource-name>, error out=w480:errorcluster)  [unwired: 2 out]
              }
            }
          }
          frame #4 {
            n250 = property on="Y Scan" class="Bool (strict)"("Val(Sgnl)"=FALSE ("Slew Ready 2")) -> ()  [unwired: 2 in, 2 out]
            n251 = property on="Y Scan Length SP steps" class="DigNum (strict)"("DisabledEnum"=T1."Enabled" ("Disabled")) -> ()  [unwired: 2 in, 2 out]
            n252 = property on="Slew Velocity" class="DigNum (strict)"("DisabledEnum"=T1."Enabled" ("Disabled")) -> ()  [unwired: 2 in, 2 out]
            n253 = property on="Scan Go" class="Bool"("DisabledEnum"=T1."Disabled and Grayed Out" ("Disabled")) -> ()  [unwired: 2 in, 2 out]
          }
        }
      }
    }
  }
  n254 = To Long Integer(number=w27) -> (32bit integer=w33:i32)
  n255 = property on="Y Step SP" class="DigNum (strict)"("Maximum"=w28) -> ()  [unwired: 2 in, 2 out]
  n256 = property on="Y Step SP" class="DigNum (strict)"("Val(Sgnl)"=w33) -> ()  [unwired: 2 in, 2 out]
  n257 = property on="Y Step SP" class="DigNum (strict)"("Minimum"=w29) -> ()  [unwired: 2 in, 2 out]
  n258 = In Range and Coerce(upper limit=w28, x=w33, lower limit=w29) -> (In Range?=w30:bool)  [unwired: 1 out]
  n259 = property on="Y in Range" class="Bool (strict)"("Val(Sgnl)"=w30) -> ()  [unwired: 2 in, 2 out]
  n260 = flat-sequence {
    tunnel: w32 -> [w497]
    tunnel: w31 -> [w494]
    frame #0 {
      n261 = call "mDrive Send Command.vi"("error in (no error)"=w494, "Command"=T2."Stop", "VISA resource name"=w497) -> ("error out"=w495:errorcluster, "VISA resource name out"=w496:refnum<visa-resource-name>)  [unwired: 4 in, 1 out]
      n262 = VISA Close(VISA resource name=w496, error in (no error)=w495) -> ()  [unwired: 1 out]
    }
  }
  "COM PORT" <- w36
  "MINPOS" <- w29
  "MAXPOS" <- w28
  "steps/rev" <- w4
  "mm/rev" <- w7
  "offset" <- 0.0 ("offset")
  "Run Current %" <- 60 ("Run Current %")
  "Holding Current %" <- 25 ("Holding Current %")
  "Backlash" <- -5120 ("Backlash2")
  "Backlash steps/sec" <- 25600 ("Value (Signaling)")
